vi "Introduce.vi"(8 "Error In":errorcluster, 11 "MedicalDroid In":refnum<class "MedicalDroid.lvclass">) -> (0 "Error Out":errorcluster, 3 "MedicalDroid Out":refnum<class "MedicalDroid.lvclass">)   [LabVIEW 2021, in "MedicalDroid.lvclass"]
doc: "Show ID of droid in prompt message for user. Comments in Polish."
uses:
  MedicalDroid.lvclass
  Read Bacta [l].vi
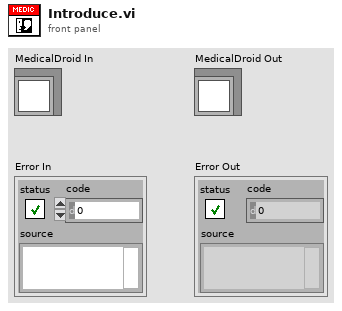
[diagram p1: front panel]
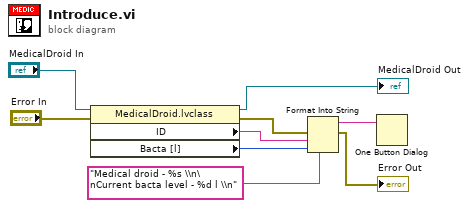
[diagram p0: block diagram]
diagram:
  n1 = property class="MedicalDroid.lvclass"(reference="MedicalDroid In", error in="Error In") -> (reference out=→"MedicalDroid Out":refnum<class "MedicalDroid.lvclass">, error out=w4:errorcluster, "ID"=w6:string, "Bacta [l]"=w5:u8)
  n2 = Format Into String(format string="Medical droid - %s \\n\nCurrent bacta level - %d l \\n", error in=w4, w6, w5) -> (resulting string=w1:string, error out=→"Error Out":errorcluster)  [unwired: 1 in]
  n3 = One Button Dialog(message=w1) -> ()  [unwired: 1 in, 1 out]
